vi "gui.default values test.vi"() -> (0 "Config Rigol DP832":T5(array[cluster])=[{"Channel"=0, "V Limit"=5.5, "I Limit"=0.5, "V Out"=5.0}, {"Channel"=1, "V Limit"=5.5, "I Limit"=0.8, "V Out"=5.0}, {"Channel"=2, "V Limit"=5.5, "I Limit"=0.2, "V Out"=0.0}] {"Channel" items=["+30V Channel 1", "+30V Channel 2", "+5V Channel 3"]}, 1 "Config Hw":T6={"VISA Rigol DP832"="USB0::0x1AB1::0x0E11::DP8C191500901::INSTR", "CTA Test#"="CTA013 A", "VISA Tek MDO3104"="USB0::0x1AB1::0x0E11::DP8C191500901::INSTR", "VISA Key 81160a"="USB0::0x1AB1::0x0E11::DP8C191500901::INSTR"}, 2 "Config VGA":T7={"Theoretical Voltage"=[0.1, 0.2, 0.3, 0.4, 0.5, 0.6, 0.7, 0.8, 0.9, 1.0], "Real Voltage"=[0.10285, 0.20714, 0.29957, 0.40485, 0.49571, 0.60685, 0.69771, 0.80114, 0.89714, 0.99885], "Pulse Width"=57344, "Frecuency Pulse"=1000000.0, "VGA Gain"=[9, 16, 24, 34, 43, 52, 61, 72, 81, 93]} {"Theoretical Voltage" format="%1.4f"; "VGA Gain" format="%02x"; "Frecuency Pulse" format="%0_2p"; "Pulse Width" format="%04x"; "Real Voltage" format="%1.5f"}, 3 "Values default":T8(array[cluster])=[{"Vsupply asic"=3.3, "Global Reset"=TRUE, "Test Register??"=TRUE, "Test ADC??"=TRUE, "Test ADC set"={"Repeats ADC"=100, "Max Desviation"=0.1}, "High ADC means"=[2.1, 1.5, 0.85, 0.1, 1.6, 1.4, 1.4, 1.3, 0.9, 2.1, 1.9], "Low ADC means"=[1.9, 1.3, 0.65, 0.0, 1.4, 1.2, 1.2, 1.1, 0.7, 1.9, 1.7], "Test MAX/MIN??"=TRUE, "Limits Max PN Min NP"={"Max P Lower"=1.888, "Min P Lower "=1.321, "Max N Lower"=1.322, "Min N Lower"=0.73, "Max P Upper"=2.177, "Min P Upper"=1.474, "Min N Upper"=0.818, "Max N Upper"=1.475}, "Test rate scan"=TRUE, "Vin Rate Scan"=[0, 1, 2, 3, 4, 5, 6, 7, 8, 9], "High rate scan"=[0.15, 0.242, 0.331, 0.425, 0.512, 0.6, 0.688, 0.774, 0.847, 0.91], "Low rate scan"=[0.021, 0.11, 0.189, 0.27, 0.347, 0.421, 0.487, 0.551, 0.601, 0.635], "Test rate scan adders??"=TRUE, "Vin Rate Adders"=[0, 1], "High rate scan add"=[0.242, 0.331, 0.425, 0.425, 0.6, 0.774], "Low rate scan add"=[0.11, 0.189, 0.27, 0.27, 0.421, 0.551], "Test offset analog??"=TRUE, "Lim Offset Analog"={"Max Analog"=0.05, "Min Analog"=-0.05}, "Test offset digital??"=TRUE, "Lim offset Dig"={"Max Dig"=0.05}, "Vsupply asic real"=38.0, "IBIAS"=TRUE, "VALUE IBIAS"=100}, {"Vsupply asic"=3.2, "Global Reset"=TRUE, "Test Register??"=TRUE, "Test ADC??"=TRUE, "Test ADC set"={"Repeats ADC"=100, "Max Desviation"=0.1}, "High ADC means"=[2.1, 1.5, 0.85, 0.1, 1.4, 1.2, 1.2, 0.7, 1.9, 0.65], "Low ADC means"=[1.9, 1.3, 0.65, 0.0, 1.6, 1.4, 1.4, 0.9, 2.1, 0.85], "Test MAX/MIN??"=TRUE, "Limits Max PN Min NP"={"Max P Lower"=1.888, "Min P Lower "=1.321, "Max N Lower"=1.322, "Min N Lower"=0.73, "Max P Upper"=2.177000045776367, "Min P Upper"=1.474, "Min N Upper"=0.818, "Max N Upper"=1.475}, "Test rate scan"=TRUE, "Vin Rate Scan"=[1, 4], "High rate scan"=[0.15, 0.242, 0.331, 0.425, 0.512, 0.6, 0.688, 0.774, 0.847, 0.91], "Low rate scan"=[0.021, 0.11, 0.189, 0.27, 0.347, 0.421, 0.487, 0.551, 0.601, 0.635], "Test rate scan adders??"=FALSE, "Vin Rate Adders"=[], "High rate scan add"=[0.15, 0.242, 0.331, 0.425, 0.512, 0.6, 0.688, 0.774, 0.847, 0.91], "Low rate scan add"=[0.021, 0.11, 0.189, 0.27, 0.347, 0.421, 0.487, 0.551, 0.601, 0.635], "Test offset analog??"=FALSE, "Lim Offset Analog"={"Max Analog"=0.05, "Min Analog"=-0.05}, "Test offset digital??"=FALSE, "Lim offset Dig"={"Max Dig"=0.05}, "Vsupply asic real"=38.0, "IBIAS"=TRUE, "VALUE IBIAS"=100}, {"Vsupply asic"=3.4, "Global Reset"=TRUE, "Test Register??"=TRUE, "Test ADC??"=TRUE, "Test ADC set"={"Repeats ADC"=100, "Max Desviation"=0.1}, "High ADC means"=[2.1, 1.5, 0.85, 0.1, 1.4, 1.2, 1.2, 0.7, 1.9, 0.65], "Low ADC means"=[1.9, 1.3, 0.65, 0.0, 1.6, 1.4, 1.4, 0.9, 2.1, 0.85], "Test MAX/MIN??"=TRUE, "Limits Max PN Min NP"={"Max P Lower"=1.888, "Min P Lower "=1.321, "Max N Lower"=1.322, "Min N Lower"=0.73, "Max P Upper"=2.177000045776367, "Min P Upper"=1.474, "Min N Upper"=0.818, "Max N Upper"=1.475}, "Test rate scan"=TRUE, "Vin Rate Scan"=[1, 4], "High rate scan"=[0.15, 0.242, 0.331, 0.425, 0.512, 0.6, 0.688, 0.774, 0.847, 0.91], "Low rate scan"=[0.021, 0.11, 0.189, 0.27, 0.347, 0.421, 0.487, 0.551, 0.601, 0.635], "Test rate scan adders??"=FALSE, "Vin Rate Adders"=[], "High rate scan add"=[0.15, 0.242, 0.331, 0.425, 0.512, 0.6, 0.688, 0.774, 0.847, 0.91], "Low rate scan add"=[0.021, 0.11, 0.189, 0.27, 0.347, 0.421, 0.487, 0.551, 0.601, 0.635], "Test offset analog??"=FALSE, "Lim Offset Analog"={"Max Analog"=0.05, "Min Analog"=-0.05}, "Test offset digital??"=FALSE, "Lim offset Dig"={"Max Dig"=0.05}, "Vsupply asic real"=38.0, "IBIAS"=TRUE, "VALUE IBIAS"=100}], 4 "Values Generator":T3[](array[typedef])=[{"Channel"=1, "Frequency"=1000000.0, "Width Time"=3.3e-09, "Amplitude"=0.05, "DC Offset"=0.0, "Load"=500.0, "Leading Edge Time"=1e-09, "Trailing Edge Time"=1e-09, "Delay"=0.0, "Out"=TRUE, "/Out"=TRUE, "Trigger Level Sync"=1, "Trigger Sync Out"=1, "Vasic Theorical"=50.0}, {"Channel"=1, "Frequency"=1000000.0, "Width Time"=3.3e-09, "Amplitude"=0.1, "DC Offset"=0.0, "Load"=500.0, "Leading Edge Time"=1e-09, "Trailing Edge Time"=1e-09, "Delay"=0.0, "Out"=TRUE, "/Out"=TRUE, "Trigger Level Sync"=1, "Trigger Sync Out"=1, "Vasic Theorical"=50.0}, {"Channel"=1, "Frequency"=1000000.0, "Width Time"=3.3e-09, "Amplitude"=0.2, "DC Offset"=0.0, "Load"=500.0, "Leading Edge Time"=1e-09, "Trailing Edge Time"=1e-09, "Delay"=0.0, "Out"=TRUE, "/Out"=TRUE, "Trigger Level Sync"=1, "Trigger Sync Out"=1, "Vasic Theorical"=50.0}, {"Channel"=1, "Frequency"=1000000.0, "Width Time"=3.3e-09, "Amplitude"=0.3, "DC Offset"=0.0, "Load"=500.0, "Leading Edge Time"=1e-09, "Trailing Edge Time"=1e-09, "Delay"=0.0, "Out"=TRUE, "/Out"=TRUE, "Trigger Level Sync"=1, "Trigger Sync Out"=1, "Vasic Theorical"=50.0}, {"Channel"=1, "Frequency"=1000000.0, "Width Time"=3.3e-09, "Amplitude"=0.4, "DC Offset"=0.0, "Load"=500.0, "Leading Edge Time"=1e-09, "Trailing Edge Time"=1e-09, "Delay"=0.0, "Out"=TRUE, "/Out"=TRUE, "Trigger Level Sync"=1, "Trigger Sync Out"=1, "Vasic Theorical"=50.0}, {"Channel"=1, "Frequency"=1000000.0, "Width Time"=3.3e-09, "Amplitude"=0.5, "DC Offset"=0.0, "Load"=500.0, "Leading Edge Time"=1e-09, "Trailing Edge Time"=1e-09, "Delay"=0.0, "Out"=TRUE, "/Out"=TRUE, "Trigger Level Sync"=1, "Trigger Sync Out"=1, "Vasic Theorical"=50.0}, {"Channel"=1, "Frequency"=1000000.0, "Width Time"=3.3e-09, "Amplitude"=0.05, "DC Offset"=0.0, "Load"=600.0, "Leading Edge Time"=1e-09, "Trailing Edge Time"=1e-09, "Delay"=0.0, "Out"=TRUE, "/Out"=TRUE, "Trigger Level Sync"=1, "Trigger Sync Out"=1, "Vasic Theorical"=50.0}, {"Channel"=1, "Frequency"=1000000.0, "Width Time"=3.3e-09, "Amplitude"=0.05, "DC Offset"=0.0, "Load"=700.0, "Leading Edge Time"=1e-09, "Trailing Edge Time"=1e-09, "Delay"=0.0, "Out"=TRUE, "/Out"=TRUE, "Trigger Level Sync"=1, "Trigger Sync Out"=1, "Vasic Theorical"=50.0}, {"Channel"=1, "Frequency"=1000000.0, "Width Time"=3.3e-09, "Amplitude"=0.05, "DC Offset"=0.0, "Load"=800.0, "Leading Edge Time"=1e-09, "Trailing Edge Time"=1e-09, "Delay"=0.0, "Out"=TRUE, "/Out"=TRUE, "Trigger Level Sync"=1, "Trigger Sync Out"=1, "Vasic Theorical"=50.0}, {"Channel"=1, "Frequency"=1000000.0, "Width Time"=3.3e-09, "Amplitude"=0.05, "DC Offset"=0.0, "Load"=900.0, "Leading Edge Time"=1e-09, "Trailing Edge Time"=1e-09, "Delay"=0.0, "Out"=TRUE, "/Out"=TRUE, "Trigger Level Sync"=1, "Trigger Sync Out"=1, "Vasic Theorical"=50.0}, {"Channel"=1, "Frequency"=1000000.0, "Width Time"=3.3e-09, "Amplitude"=0.05, "DC Offset"=0.0, "Load"=1000.0, "Leading Edge Time"=1e-09, "Trailing Edge Time"=1e-09, "Delay"=0.0, "Out"=TRUE, "/Out"=TRUE, "Trigger Level Sync"=1, "Trigger Sync Out"=1, "Vasic Theorical"=50.0}] {"Vasic Theorical" min=1.0 max=1000000.0 step=1.0 format="%#_6pV"; "Frequency" min=0.001 max=333000000.0 step=1000.0 format="%#_6pHz"; "Leading Edge Time" min=1e-09 max=1.0 step=1e-10 format="%#_6ps"; "Trailing Edge Time" min=1e-09 max=1.0 step=1e-10 format="%#_6ps"; "Delay" min=0.0 max=1.0 step=1e-12 format="%#_6ps"; "Trigger Level Sync" items=["ECL", "TTL"]; "Trigger Sync Out" items=["AB"=3, "B"=2, "A"=1, "None"=0]; "Load" min=1.0 max=1000000.0 step=1.0 format="%#_6p"; "DC Offset" min=-10.0 max=10.0 step=0.1 format="%#_6pV"; "Amplitude" min=0.05 max=5.0 step=0.001 format="%#_6pV"; "Width Time" min=1.5e-09 max=1.0 step=1e-10 format="%#_6ps"; "Channel" items=["Channel1"=1, "Channel2"=2]})   [LabVIEW 2019]
uses:
  TEST.TEST CONFIG VGA.ctl
  Rigol DP832/DP832_Control Channels.ctl
  GenPulse_configurar.ctl
  TEST.TEST CONFIG TEST MATRIZ.ctl
  TEST.TEST CONFIG TEST.ctl
panel:
  in  "Config Test":T1=[{"Vasic"=2.8, "Global Reset"=FALSE, "Test Register?"=FALSE, "Test ADC?"=FALSE, "Test ADC"={"Repeats ADC"=100, "Max Desviation"=0.1}, "Limits ADC"={"Low"=[1.9, 1.3, 0.65, 0.0, 1.6, 1.4, 1.4, 0.9, 2.1, 0.85, 1.9], "High"=[2.1, 1.5, 0.85, 0.1, 1.4, 1.2, 1.2, 0.7, 1.9, 0.65, 1.7]}, "Test Max PN Min NP?"=FALSE, "Limits Max PN Min NP"={"Max P Upper"=2.177000045776367, "Min P Upper"=1.474, "Max N Upper"=1.475, "Min N Upper"=0.818, "Max P Lower"=1.888, "Min P Lower "=1.321, "Max N Lower"=1.322, "Min N Lower"=0.73}, "Test Rate Scan?"=FALSE, "Vin Rate Scan"=[], "Limits Rate Scan"={"High"=[0.15, 0.242, 0.331, 0.425, 0.512, 0.6, 0.688, 0.774, 0.847, 0.91], "Low"=[0.021, 0.11, 0.189, 0.27, 0.347, 0.421, 0.487, 0.551, 0.601, 0.635]}, "Test Rate Scan Adders?"=FALSE, "Vin Rate Adders"=[], "Limits Rate Scan adders"={"High"=[], "Low"=[]}, "Test offset analog?"=FALSE, "Lim Offset Analog"={"Max Analog"=0.05, "Min Analog"=-0.05}, "Test offset digital?"=FALSE, "Lim offset Dig"={"Max Dig"=0.05}, "Vasic real f.a."=2.8, "IBIAS"=FALSE, "VALUE IBIAS"=63}, {"Vasic"=2.8, "Global Reset"=FALSE, "Test Register?"=FALSE, "Test ADC?"=FALSE, "Test ADC"={"Repeats ADC"=100, "Max Desviation"=0.1}, "Limits ADC"={"Low"=[1.9, 1.3, 0.65, 0.0, 1.6, 1.4, 1.4, 0.9, 2.1, 0.85, 1.9], "High"=[2.1, 1.5, 0.85, 0.1, 1.4, 1.2, 1.2, 0.7, 1.9, 0.65, 1.7]}, "Test Max PN Min NP?"=FALSE, "Limits Max PN Min NP"={"Max P Upper"=2.177000045776367, "Min P Upper"=1.474, "Max N Upper"=1.475, "Min N Upper"=0.818, "Max P Lower"=1.888, "Min P Lower "=1.321, "Max N Lower"=1.322, "Min N Lower"=0.73}, "Test Rate Scan?"=FALSE, "Vin Rate Scan"=[], "Limits Rate Scan"={"High"=[0.15, 0.242, 0.331, 0.425, 0.512, 0.6, 0.688, 0.774, 0.847, 0.91], "Low"=[0.021, 0.11, 0.189, 0.27, 0.347, 0.421, 0.487, 0.551, 0.601, 0.635]}, "Test Rate Scan Adders?"=FALSE, "Vin Rate Adders"=[], "Limits Rate Scan adders"={"High"=[], "Low"=[]}, "Test offset analog?"=FALSE, "Lim Offset Analog"={"Max Analog"=0.05, "Min Analog"=-0.05}, "Test offset digital?"=FALSE, "Lim offset Dig"={"Max Dig"=0.05}, "Vasic real f.a."=2.8, "IBIAS"=FALSE, "VALUE IBIAS"=63}, {"Vasic"=2.8, "Global Reset"=FALSE, "Test Register?"=FALSE, "Test ADC?"=FALSE, "Test ADC"={"Repeats ADC"=100, "Max Desviation"=0.1}, "Limits ADC"={"Low"=[1.9, 1.3, 0.65, 0.0, 1.6, 1.4, 1.4, 0.9, 2.1, 0.85, 1.9], "High"=[2.1, 1.5, 0.85, 0.1, 1.4, 1.2, 1.2, 0.7, 1.9, 0.65, 1.7]}, "Test Max PN Min NP?"=FALSE, "Limits Max PN Min NP"={"Max P Upper"=2.177000045776367, "Min P Upper"=1.474, "Max N Upper"=1.475, "Min N Upper"=0.818, "Max P Lower"=1.888, "Min P Lower "=1.321, "Max N Lower"=1.322, "Min N Lower"=0.73}, "Test Rate Scan?"=FALSE, "Vin Rate Scan"=[], "Limits Rate Scan"={"High"=[0.15, 0.242, 0.331, 0.425, 0.512, 0.6, 0.688, 0.774, 0.847, 0.91], "Low"=[0.021, 0.11, 0.189, 0.27, 0.347, 0.421, 0.487, 0.551, 0.601, 0.635]}, "Test Rate Scan Adders?"=FALSE, "Vin Rate Adders"=[], "Limits Rate Scan adders"={"High"=[], "Low"=[]}, "Test offset analog?"=FALSE, "Lim Offset Analog"={"Max Analog"=0.05, "Min Analog"=-0.05}, "Test offset digital?"=FALSE, "Lim offset Dig"={"Max Dig"=0.05}, "Vasic real f.a."=2.8, "IBIAS"=FALSE, "VALUE IBIAS"=63}, {"Vasic"=2.8, "Global Reset"=FALSE, "Test Register?"=FALSE, "Test ADC?"=FALSE, "Test ADC"={"Repeats ADC"=100, "Max Desviation"=0.1}, "Limits ADC"={"Low"=[1.9, 1.3, 0.65, 0.0, 1.6, 1.4, 1.4, 0.9, 2.1, 0.85, 1.9], "High"=[2.1, 1.5, 0.85, 0.1, 1.4, 1.2, 1.2, 0.7, 1.9, 0.65, 1.7]}, "Test Max PN Min NP?"=FALSE, "Limits Max PN Min NP"={"Max P Upper"=2.177000045776367, "Min P Upper"=1.474, "Max N Upper"=1.475, "Min N Upper"=0.818, "Max P Lower"=1.888, "Min P Lower "=1.321, "Max N Lower"=1.322, "Min N Lower"=0.73}, "Test Rate Scan?"=FALSE, "Vin Rate Scan"=[], "Limits Rate Scan"={"High"=[0.15, 0.242, 0.331, 0.425, 0.512, 0.6, 0.688, 0.774, 0.847, 0.91], "Low"=[0.021, 0.11, 0.189, 0.27, 0.347, 0.421, 0.487, 0.551, 0.601, 0.635]}, "Test Rate Scan Adders?"=FALSE, "Vin Rate Adders"=[], "Limits Rate Scan adders"={"High"=[], "Low"=[]}, "Test offset analog?"=FALSE, "Lim Offset Analog"={"Max Analog"=0.05, "Min Analog"=-0.05}, "Test offset digital?"=FALSE, "Lim offset Dig"={"Max Dig"=0.05}, "Vasic real f.a."=2.8, "IBIAS"=FALSE, "VALUE IBIAS"=63}] {"VALUE IBIAS" max=63 step=1; "Vasic real f.a." min=2.8 max=3.8 step=0.01 format="%.2g"; "Limits Rate Scan adders"."Low" format="%1.3f"; "Limits Rate Scan adders"."High" format="%1.3f"; "Limits ADC"."High" format="%1.4f"; "Limits ADC"."Low" format="%1.3f"; "Lim offset Dig"."Max Dig" format="%.3g"; "Lim Offset Analog"."Min Analog" format="%.3g"; "Lim Offset Analog"."Max Analog" format="%.3g"; "Limits Rate Scan"."Low" format="%1.4f"; "Limits Rate Scan"."High" format="%1.3f"; "Limits Max PN Min NP"."Min P Upper" format="%.3g"; "Limits Max PN Min NP"."Min P Lower" format="%.3g"; "Limits Max PN Min NP"."Max N Lower" format="%.3g"; "Limits Max PN Min NP"."Max N Upper" format="%.3g"; "Limits Max PN Min NP"."Min N Lower" format="%.3g"; "Limits Max PN Min NP"."Min N Upper" format="%.3g"; "Limits Max PN Min NP"."Max P Upper" format="%.3g"; "Limits Max PN Min NP"."Max P Lower" format="%.3g"; "Vasic" min=2.8 max=3.8 step=0.01 format="%.2g"}
  # "Modo 2\nModo 3\nModo 4\nModo 2\nModo 3\nModo 4"
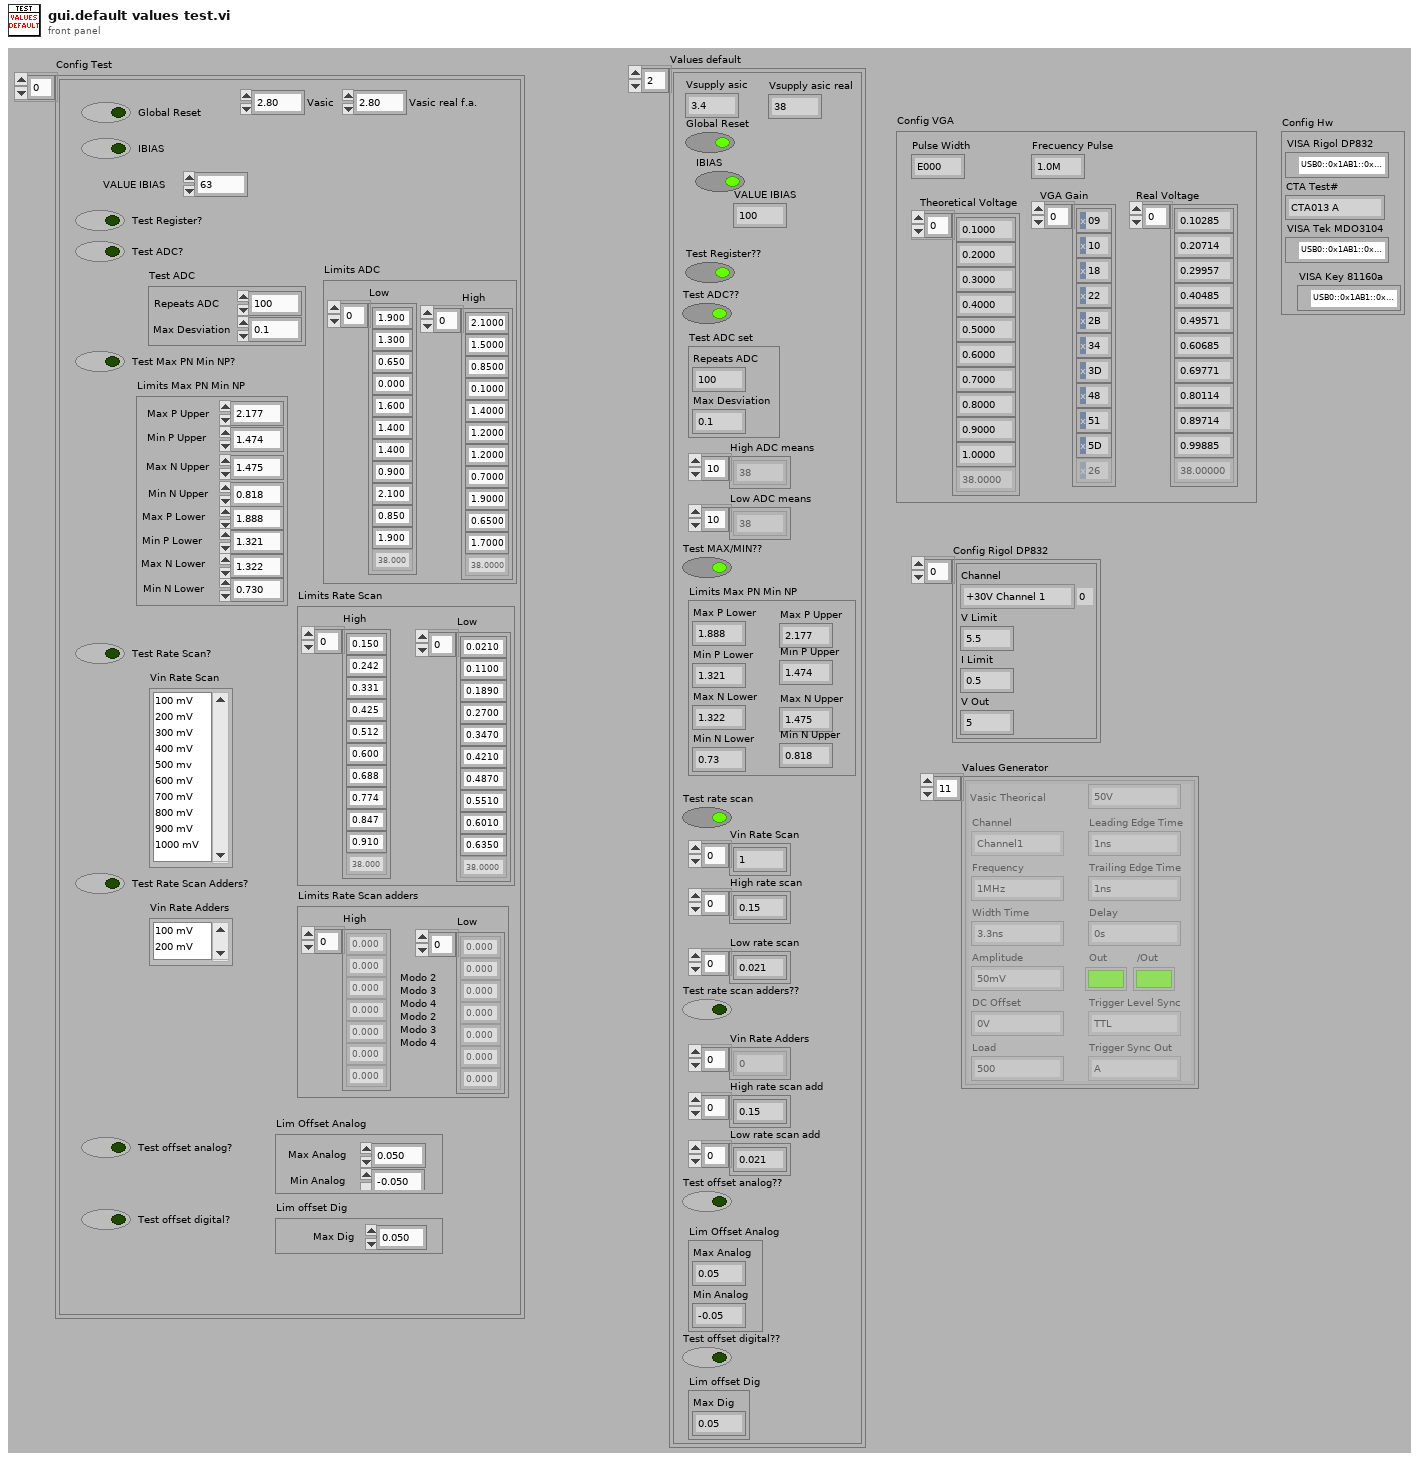
[diagram p1: front panel]
types:
  T1 = typedef "TEST.TEST CONFIG TEST MATRIZ.ctl" = T2[]
  T2 = typedef "TEST.TEST CONFIG TEST.ctl" = cluster{"Vasic":dbl, "Global Reset":bool, "Test Register?":bool, "Test ADC?":bool, "Test ADC":cluster{"Repeats ADC":i32, "Max Desviation":dbl}, "Limits ADC":cluster{"Low":dbl[], "High":dbl[]}, "Test Max PN Min NP?":bool, "Limits Max PN Min NP":cluster{"Max P Upper":dbl, "Min P Upper":dbl, "Max N Upper":dbl, "Min N Upper":dbl, "Max P Lower":dbl, "Min P Lower ":dbl, "Max N Lower":dbl, "Min N Lower":dbl}, "Test Rate Scan?":bool, "Vin Rate Scan":i32[], "Limits Rate Scan":cluster{"High":dbl[], "Low":dbl[]}, "Test Rate Scan Adders?":bool, "Vin Rate Adders":i32[], "Limits Rate Scan adders":cluster{"High":dbl[], "Low":dbl[]}, "Test offset analog?":bool, "Lim Offset Analog":cluster{"Max Analog":dbl, "Min Analog":dbl}, "Test offset digital?":bool, "Lim offset Dig":cluster{"Max Dig":dbl}, "Vasic real f.a.":dbl, "IBIAS":bool, "VALUE IBIAS":u8}
  T3 = typedef "GenPulse_configurar.ctl" = cluster{"Channel":u16, "Frequency":dbl, "Width Time":dbl, "Amplitude":dbl, "DC Offset":dbl, "Load":dbl, "Leading Edge Time":dbl, "Trailing Edge Time":dbl, "Delay":dbl, "Out":bool, "/Out":bool, "Trigger Level Sync":u16, "Trigger Sync Out":u16, "Vasic Theorical":dbl}
  T4 = typedef "DP832_Control Channels.ctl" = i32
  T5 = cluster{"Channel":T4, "V Limit":dbl, "I Limit":dbl, "V Out":dbl}[]
  T6 = cluster{"VISA Rigol DP832":refnum<visa-resource-name>, "CTA Test#":string, "VISA Tek MDO3104":refnum<visa-resource-name>, "VISA Key 81160a":refnum<visa-resource-name>}
  T7 = typedef "TEST.TEST CONFIG VGA.ctl" = cluster{"Theoretical Voltage":dbl[], "Real Voltage":dbl[], "Pulse Width":u16, "Frecuency Pulse":dbl, "VGA Gain":u8[]}
  T8 = cluster{"Vsupply asic":dbl, "Global Reset":bool, "Test Register??":bool, "Test ADC??":bool, "Test ADC set":cluster{"Repeats ADC":i32, "Max Desviation":dbl}, "High ADC means":dbl[], "Low ADC means":dbl[], "Test MAX/MIN??":bool, "Limits Max PN Min NP":cluster{"Max P Lower":dbl, "Min P Lower ":dbl, "Max N Lower":dbl, "Min N Lower":dbl, "Max P Upper":dbl, "Min P Upper":dbl, "Min N Upper":dbl, "Max N Upper":dbl}, "Test rate scan":bool, "Vin Rate Scan":i32[], "High rate scan":dbl[], "Low rate scan":dbl[], "Test rate scan adders??":bool, "Vin Rate Adders":i32[], "High rate scan add":dbl[], "Low rate scan add":dbl[], "Test offset analog??":bool, "Lim Offset Analog":cluster{"Max Analog":dbl, "Min Analog":dbl}, "Test offset digital??":bool, "Lim offset Dig":cluster{"Max Dig":dbl}, "Vsupply asic real":dbl, "IBIAS":bool, "VALUE IBIAS":u8}[]
  T9 = cluster{"Vsupply asic":dbl, "Global Reset":bool, "Test register??":bool, "Test ADC??":bool, "Test ADC set":cluster{"Repeats ADC":i32, "Max Desviation":dbl}, "High ADC means":dbl[], "Low ADC means":dbl[], "Test MAX/MIN??":bool, "Limits Max PN Min NP":cluster{"Max P Lower":dbl, "Min P Lower ":dbl, "Max N Lower":dbl, "Min N Lower":dbl, "Max P Upper":dbl, "Min P Upper":dbl, "Min N Upper":dbl, "Max N Upper":dbl}, "Test rate scan":bool, "Vin Rate Scan":i32[], "High rate scan":dbl[], "Low rate scan":dbl[], "Test rate scan adders??":bool, "Vin Rate Adders":i32[], "High rate scan add":dbl[], "Low rate scan add":dbl[], "Test offset analog??":bool, "Lim Offset Analog":cluster{"Max Analog":dbl, "Min Analog":dbl}, "Test offset digital??":bool, "Lim offset Dig":cluster{"Max Dig":dbl}, "Vsupply asic REAL":dbl, "IBIAS":bool, "VALUE IBIAS":u8}[]
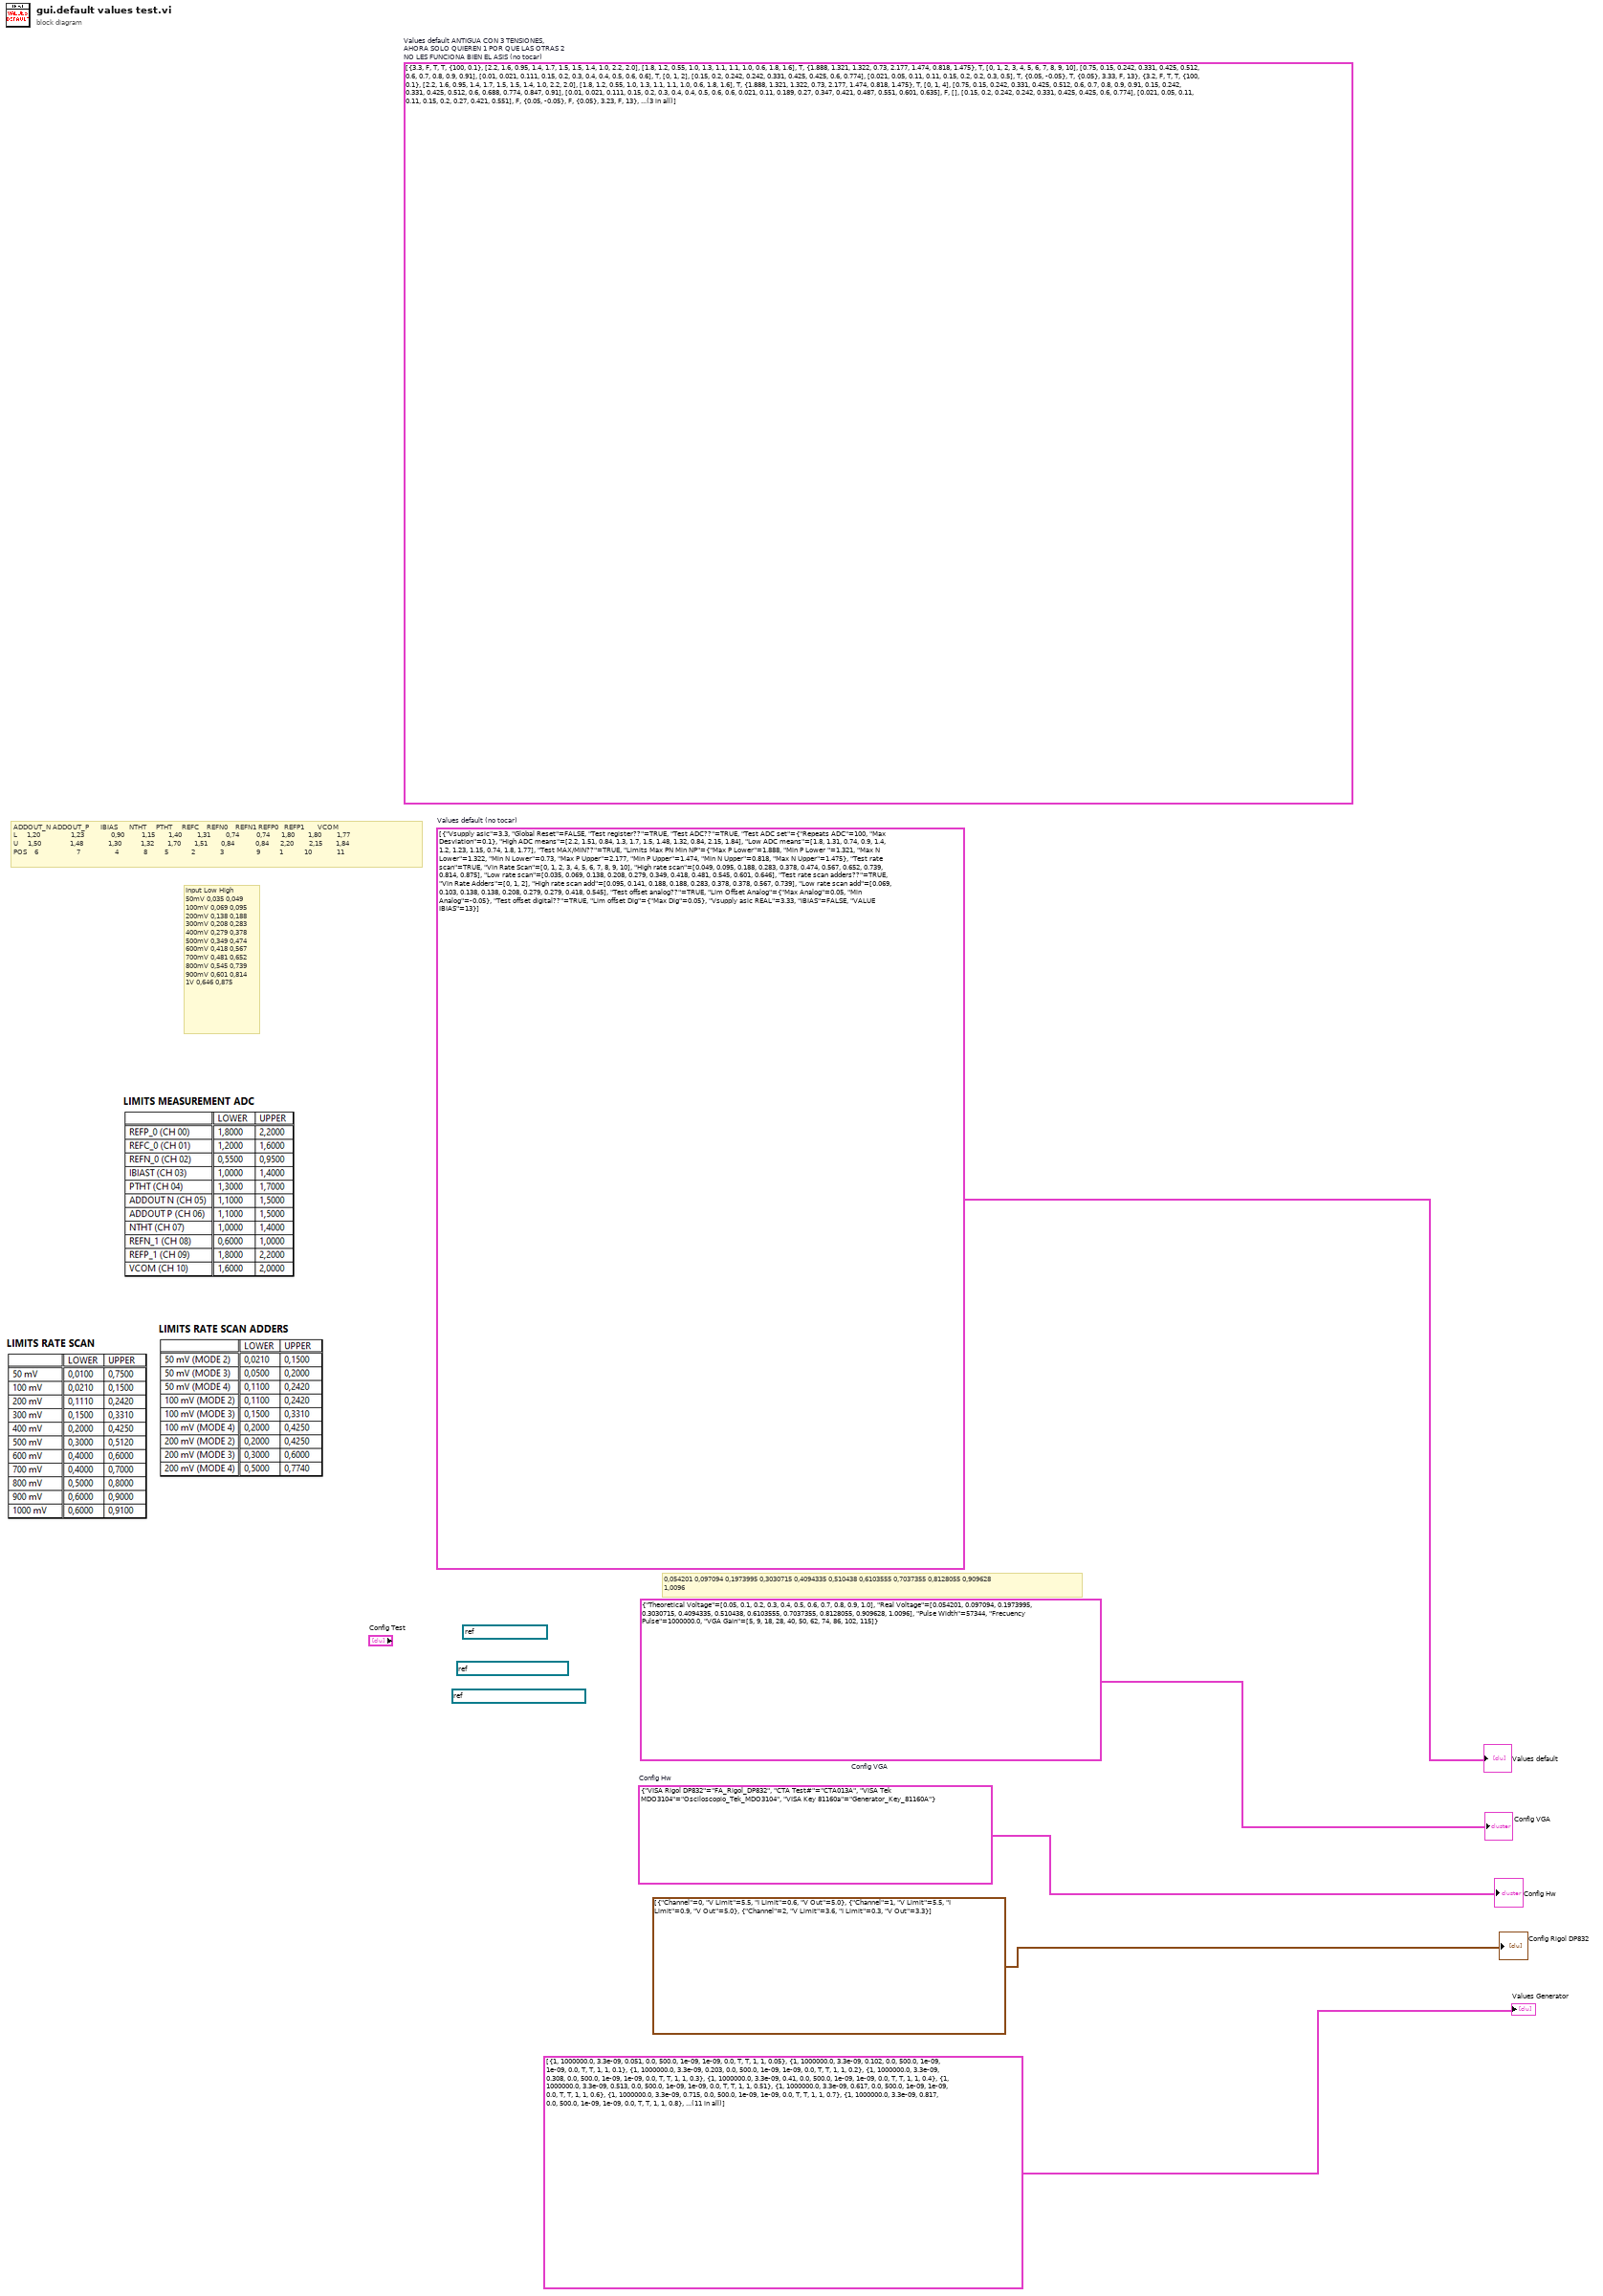
[diagram p0: block diagram]
diagram:
  (unwired) T9 [{"Vsupply asic"=3.3, "Global Reset"=FALSE, "Test register??"=TRUE, "Test ADC??"=TRUE, "Test ADC set"={"Repeats ADC"=100, "Max Desviation"=0.1}, "High ADC means"=[2.2, 1.6, 0.95, 1.4, 1.7, 1.5, 1.5, 1.4, 1.0, 2.2, 2.0], "Low ADC means"=[1.8, 1.2, 0.55, 1.0, 1.3, 1.1, 1.1, 1.0, 0.6, 1.8, 1.6], "Test MAX/MIN??"=TRUE, "Limits Max PN Min NP"={"Max P Lower"=1.888, "Min P Lower "=1.321, "Max N Lower"=1.322, "Min N Lower"=0.73, "Max P Upper"=2.177, "Min P Upper"=1.474, "Min N Upper"=0.818, "Max N Upper"=1.475}, "Test rate scan"=TRUE, "Vin Rate Scan"=[0, 1, 2, 3, 4, 5, 6, 7, 8, 9, 10], "High rate scan"=[0.75, 0.15, 0.242, 0.331, 0.425, 0.512, 0.6, 0.7, 0.8, 0.9, 0.91], "Low rate scan"=[0.01, 0.021, 0.111, 0.15, 0.2, 0.3, 0.4, 0.4, 0.5, 0.6, 0.6], "Test rate scan adders??"=TRUE, "Vin Rate Adders"=[0, 1, 2], "High rate scan add"=[0.15, 0.2, 0.242, 0.242, 0.331, 0.425, 0.425, 0.6, 0.774], "Low rate scan add"=[0.021, 0.05, 0.11, 0.11, 0.15, 0.2, 0.2, 0.3, 0.5], "Test offset analog??"=TRUE, "Lim Offset Analog"={"Max Analog"=0.05, "Min Analog"=-0.05}, "Test offset digital??"=TRUE, "Lim offset Dig"={"Max Dig"=0.05}, "Vsupply asic REAL"=3.33, "IBIAS"=FALSE, "VALUE IBIAS"=13}, {"Vsupply asic"=3.2, "Global Reset"=FALSE, "Test register??"=TRUE, "Test ADC??"=TRUE, "Test ADC set"={"Repeats ADC"=100, "Max Desviation"=0.1}, "High ADC means"=[2.2, 1.6, 0.95, 1.4, 1.7, 1.5, 1.5, 1.4, 1.0, 2.2, 2.0], "Low ADC means"=[1.8, 1.2, 0.55, 1.0, 1.3, 1.1, 1.1, 1.0, 0.6, 1.8, 1.6], "Test MAX/MIN??"=TRUE, "Limits Max PN Min NP"={"Max P Lower"=1.888, "Min P Lower "=1.321, "Max N Lower"=1.322, "Min N Lower"=0.73, "Max P Upper"=2.177, "Min P Upper"=1.474, "Min N Upper"=0.818, "Max N Upper"=1.475}, "Test rate scan"=TRUE, "Vin Rate Scan"=[0, 1, 4], "High rate scan"=[0.75, 0.15, 0.242, 0.331, 0.425, 0.512, 0.6, 0.7, 0.8, 0.9, 0.91, 0.15, 0.242, 0.331, 0.425, 0.512, 0.6, 0.688, 0.774, 0.847, 0.91], "Low rate scan"=[0.01, 0.021, 0.111, 0.15, 0.2, 0.3, 0.4, 0.4, 0.5, 0.6, 0.6, 0.021, 0.11, 0.189, 0.27, 0.347, 0.421, 0.487, 0.551, 0.601, 0.635], "Test rate scan adders??"=FALSE, "Vin Rate Adders"=[], "High rate scan add"=[0.15, 0.2, 0.242, 0.242, 0.331, 0.425, 0.425, 0.6, 0.774], "Low rate scan add"=[0.021, 0.05, 0.11, 0.11, 0.15, 0.2, 0.27, 0.421, 0.551], "Test offset analog??"=FALSE, "Lim Offset Analog"={"Max Analog"=0.05, "Min Analog"=-0.05}, "Test offset digital??"=FALSE, "Lim offset Dig"={"Max Dig"=0.05}, "Vsupply asic REAL"=3.23, "IBIAS"=FALSE, "VALUE IBIAS"=13}, {"Vsupply asic"=3.4, "Global Reset"=FALSE, "Test register??"=TRUE, "Test ADC??"=TRUE, "Test ADC set"={"Repeats ADC"=100, "Max Desviation"=0.1}, "High ADC means"=[2.2, 1.6, 0.95, 1.4, 1.7, 1.5, 1.5, 1.4, 1.0, 2.2, 2.0], "Low ADC means"=[1.8, 1.2, 0.55, 1.0, 1.3, 1.1, 1.1, 1.0, 0.6, 1.8, 1.6], "Test MAX/MIN??"=TRUE, "Limits Max PN Min NP"={"Max P Lower"=1.888, "Min P Lower "=1.321, "Max N Lower"=1.322, "Min N Lower"=0.73, "Max P Upper"=2.177, "Min P Upper"=1.474, "Min N Upper"=0.818, "Max N Upper"=1.475}, "Test rate scan"=TRUE, "Vin Rate Scan"=[0, 1, 4], "High rate scan"=[0.75, 0.15, 0.242, 0.331, 0.425, 0.512, 0.6, 0.7, 0.8, 0.9, 0.91], "Low rate scan"=[0.01, 0.021, 0.111, 0.15, 0.2, 0.3, 0.4, 0.4, 0.5, 0.6, 0.6], "Test rate scan adders??"=FALSE, "Vin Rate Adders"=[], "High rate scan add"=[0.15, 0.2, 0.242, 0.242, 0.331, 0.425, 0.425, 0.6, 0.774], "Low rate scan add"=[0.021, 0.05, 0.11, 0.11, 0.15, 0.2, 0.27, 0.421, 0.551], "Test offset analog??"=FALSE, "Lim Offset Analog"={"Max Analog"=0.05, "Min Analog"=-0.05}, "Test offset digital??"=FALSE, "Lim offset Dig"={"Max Dig"=0.05}, "Vsupply asic REAL"=3.43, "IBIAS"=FALSE, "VALUE IBIAS"=13}]  # Values default ANTIGUA CON 3 TENSIONES, AHORA SOLO QUIEREN 1 POR QUE LAS OTRAS 2 NO LES FUNCIONA BIEN EL ASIS (no tocar)
  (unwired) refnum<visa-resource-name> "Osciloscopio_Tek_MDO3104" ("VISA resource name 3")
  (unwired) refnum<visa-resource-name> "Generator_Key_81160A" ("VISA resource name 2")
  (unwired) refnum<visa-resource-name> "FA_Rigol_DP832" ("VISA resource name")
  w3 = T6 {"VISA Rigol DP832"="FA_Rigol_DP832", "CTA Test#"="CTA013A", "VISA Tek MDO3104"="Osciloscopio_Tek_MDO3104", "VISA Key 81160a"="Generator_Key_81160A"}  # Config Hw
  w4 = T7 {"Theoretical Voltage"=[0.05, 0.1, 0.2, 0.3, 0.4, 0.5, 0.6, 0.7, 0.8, 0.9, 1.0], "Real Voltage"=[0.054201, 0.097094, 0.1973995, 0.3030715, 0.4094335, 0.510438, 0.6103555, 0.7037355, 0.8128055, 0.909628, 1.0096], "Pulse Width"=57344, "Frecuency Pulse"=1000000.0, "VGA Gain"=[5, 9, 18, 28, 40, 50, 62, 74, 86, 102, 115]}  # Config VGA
  w5 = T9 [{"Vsupply asic"=3.3, "Global Reset"=FALSE, "Test register??"=TRUE, "Test ADC??"=TRUE, "Test ADC set"={"Repeats ADC"=100, "Max Desviation"=0.1}, "High ADC means"=[2.2, 1.51, 0.84, 1.3, 1.7, 1.5, 1.48, 1.32, 0.84, 2.15, 1.84], "Low ADC means"=[1.8, 1.31, 0.74, 0.9, 1.4, 1.2, 1.23, 1.15, 0.74, 1.8, 1.77], "Test MAX/MIN??"=TRUE, "Limits Max PN Min NP"={"Max P Lower"=1.888, "Min P Lower "=1.321, "Max N Lower"=1.322, "Min N Lower"=0.73, "Max P Upper"=2.177, "Min P Upper"=1.474, "Min N Upper"=0.818, "Max N Upper"=1.475}, "Test rate scan"=TRUE, "Vin Rate Scan"=[0, 1, 2, 3, 4, 5, 6, 7, 8, 9, 10], "High rate scan"=[0.049, 0.095, 0.188, 0.283, 0.378, 0.474, 0.567, 0.652, 0.739, 0.814, 0.875], "Low rate scan"=[0.035, 0.069, 0.138, 0.208, 0.279, 0.349, 0.418, 0.481, 0.545, 0.601, 0.646], "Test rate scan adders??"=TRUE, "Vin Rate Adders"=[0, 1, 2], "High rate scan add"=[0.095, 0.141, 0.188, 0.188, 0.283, 0.378, 0.378, 0.567, 0.739], "Low rate scan add"=[0.069, 0.103, 0.138, 0.138, 0.208, 0.279, 0.279, 0.418, 0.545], "Test offset analog??"=TRUE, "Lim Offset Analog"={"Max Analog"=0.05, "Min Analog"=-0.05}, "Test offset digital??"=TRUE, "Lim offset Dig"={"Max Dig"=0.05}, "Vsupply asic REAL"=3.33, "IBIAS"=FALSE, "VALUE IBIAS"=13}]  # Values default (no tocar)
  # "ADDOUT_N\tADDOUT_P\t     IBIAS     \tNTHT    \tPTHT    \tREFC   \tREFN0\t   REFN1\tREFP0  \tREFP1\t      VCOM\nL    \t1,20                1,23\t             0,90        \t1,15      \t1,40\t       1,31\t       0,74\t        0,74\t     1,80\t      1,80\t       1,77\nU\t    1,50               1,48\t            1,30         \t1,32  \t    1,70  \t    1,51\t      0,84          \t0,84\t     2,20\t       2,15      \t1,84\nPOS    6                    7                  4             8         5            2             3                 9          1           10             11"
  # "Input\tLow\tHigh\n50mV\t0,035\t0,049\n100mV\t0,069\t0,095\n200mV\t0,138\t0,188\n300mV\t0,208\t0,283\n400mV\t0,279\t0,378\n500mV\t0,349\t0,474\n600mV\t0,418\t0,567\n700mV\t0,481\t0,652\n800mV\t0,545\t0,739\n900mV\t0,601\t0,814\n1V\t0,646\t0,875"
  # "0,054201\t0,097094\t0,1973995\t0,3030715\t0,4094335\t0,510438\t0,6103555\t0,7037355\t0,8128055\t0,909628\t1,0096"
  "Values default" <- w5
  "Config VGA" <- w4
  "Config Hw" <- w3
  "Config Rigol DP832" <- T5 [{"Channel"=0, "V Limit"=5.5, "I Limit"=0.6, "V Out"=5.0}, {"Channel"=1, "V Limit"=5.5, "I Limit"=0.9, "V Out"=5.0}, {"Channel"=2, "V Limit"=3.6, "I Limit"=0.3, "V Out"=3.3}] ("Config Rigol DP832")
  "Values Generator" <- T3[] [{"Channel"=1, "Frequency"=1000000.0, "Width Time"=3.3e-09, "Amplitude"=0.051, "DC Offset"=0.0, "Load"=500.0, "Leading Edge Time"=1e-09, "Trailing Edge Time"=1e-09, "Delay"=0.0, "Out"=TRUE, "/Out"=TRUE, "Trigger Level Sync"=1, "Trigger Sync Out"=1, "Vasic Theorical"=0.05}, {"Channel"=1, "Frequency"=1000000.0, "Width Time"=3.3e-09, "Amplitude"=0.102, "DC Offset"=0.0, "Load"=500.0, "Leading Edge Time"=1e-09, "Trailing Edge Time"=1e-09, "Delay"=0.0, "Out"=TRUE, "/Out"=TRUE, "Trigger Level Sync"=1, "Trigger Sync Out"=1, "Vasic Theorical"=0.1}, {"Channel"=1, "Frequency"=1000000.0, "Width Time"=3.3e-09, "Amplitude"=0.203, "DC Offset"=0.0, "Load"=500.0, "Leading Edge Time"=1e-09, "Trailing Edge Time"=1e-09, "Delay"=0.0, "Out"=TRUE, "/Out"=TRUE, "Trigger Level Sync"=1, "Trigger Sync Out"=1, "Vasic Theorical"=0.2}, {"Channel"=1, "Frequency"=1000000.0, "Width Time"=3.3e-09, "Amplitude"=0.308, "DC Offset"=0.0, "Load"=500.0, "Leading Edge Time"=1e-09, "Trailing Edge Time"=1e-09, "Delay"=0.0, "Out"=TRUE, "/Out"=TRUE, "Trigger Level Sync"=1, "Trigger Sync Out"=1, "Vasic Theorical"=0.3}, {"Channel"=1, "Frequency"=1000000.0, "Width Time"=3.3e-09, "Amplitude"=0.41, "DC Offset"=0.0, "Load"=500.0, "Leading Edge Time"=1e-09, "Trailing Edge Time"=1e-09, "Delay"=0.0, "Out"=TRUE, "/Out"=TRUE, "Trigger Level Sync"=1, "Trigger Sync Out"=1, "Vasic Theorical"=0.4}, {"Channel"=1, "Frequency"=1000000.0, "Width Time"=3.3e-09, "Amplitude"=0.513, "DC Offset"=0.0, "Load"=500.0, "Leading Edge Time"=1e-09, "Trailing Edge Time"=1e-09, "Delay"=0.0, "Out"=TRUE, "/Out"=TRUE, "Trigger Level Sync"=1, "Trigger Sync Out"=1, "Vasic Theorical"=0.51}, {"Channel"=1, "Frequency"=1000000.0, "Width Time"=3.3e-09, "Amplitude"=0.617, "DC Offset"=0.0, "Load"=500.0, "Leading Edge Time"=1e-09, "Trailing Edge Time"=1e-09, "Delay"=0.0, "Out"=TRUE, "/Out"=TRUE, "Trigger Level Sync"=1, "Trigger Sync Out"=1, "Vasic Theorical"=0.6}, {"Channel"=1, "Frequency"=1000000.0, "Width Time"=3.3e-09, "Amplitude"=0.715, "DC Offset"=0.0, "Load"=500.0, "Leading Edge Time"=1e-09, "Trailing Edge Time"=1e-09, "Delay"=0.0, "Out"=TRUE, "/Out"=TRUE, "Trigger Level Sync"=1, "Trigger Sync Out"=1, "Vasic Theorical"=0.7}, {"Channel"=1, "Frequency"=1000000.0, "Width Time"=3.3e-09, "Amplitude"=0.817, "DC Offset"=0.0, "Load"=500.0, "Leading Edge Time"=1e-09, "Trailing Edge Time"=1e-09, "Delay"=0.0, "Out"=TRUE, "/Out"=TRUE, "Trigger Level Sync"=1, "Trigger Sync Out"=1, "Vasic Theorical"=0.8}, {"Channel"=1, "Frequency"=1000000.0, "Width Time"=3.3e-09, "Amplitude"=0.919, "DC Offset"=0.0, "Load"=500.0, "Leading Edge Time"=1e-09, "Trailing Edge Time"=1e-09, "Delay"=0.0, "Out"=TRUE, "/Out"=TRUE, "Trigger Level Sync"=1, "Trigger Sync Out"=1, "Vasic Theorical"=0.9}, {"Channel"=1, "Frequency"=1000000.0, "Width Time"=3.3e-09, "Amplitude"=1.022, "DC Offset"=0.0, "Load"=500.0, "Leading Edge Time"=1e-09, "Trailing Edge Time"=1e-09, "Delay"=0.0, "Out"=TRUE, "/Out"=TRUE, "Trigger Level Sync"=1, "Trigger Sync Out"=1, "Vasic Theorical"=1.0}]
